vi "eventHardpointActuatorInfo.vi"(8 "error in (no error)":errorcluster, 11 "Publisher in":refnum<class "Publisher.lvclass">) -> (0 "error out":errorcluster, 3 "Publisher out":refnum<class "Publisher.lvclass">)   [LabVIEW 2016, in "Publisher.lvclass"]
uses:
  Publisher.lvclass
  Publisher.lvclass/Publisher.ctl
  UserEvents/UserEvents.lvclass
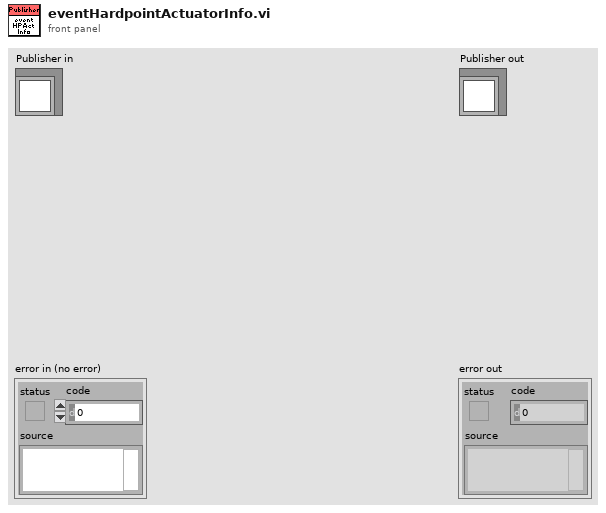
[diagram p1: front panel]
types:
  T1 = typedef "M1M3SupportTopics.lvlib/EventHardpointActuatorInfo.ctl" = cluster{"Timestamp":T2, "ReferenceId":i32[], "ReferencePosition":i32[], "XPosition":sgl[], "YPosition":sgl[], "ZPosition":sgl[], "ILCUniqueId":i64[], "ILCApplicationType":u8[], "NetworkNodeType":u8[], "ILCSelectedOptions":u8[], "NetworkNodeOptions":u8[], "MajorRevision":u8[], "MinorRevision":u8[], "ADCScanRate":u8[], "MainADCCalibrationK1":sgl[], "MainADCCalibrationK2":sgl[], "MainADCCalibrationK3":sgl[], "MainADCCalibrationK4":sgl[], "MainLoadCellOffset":sgl[], "MainLoadCellSensitivity":sgl[], "BackupADCCalibrationK1":sgl[], "BackupADCCalibrationK2":sgl[], "BackupADCCalibrationK3":sgl[], "BackupADCCalibrationK4":sgl[], "BackupLoadCellOffset":sgl[], "BackupLoadCellSensitivity":sgl[], "MainCalibrationError":bool[], "BackupCalibrationError":bool[], "UniqueIdCRCError":bool[], "ApplicationTypeMismatch":bool[], "ApplicationMissing":bool[], "ApplicationCRCMismatch":bool[], "OneWireMissing":bool[], "OneWire1Mismatch":bool[], "OneWire2Mismatch":bool[]}
  T2 = typedef "M1M3SupportTopics.lvlib/Timestamp.ctl" = dbl
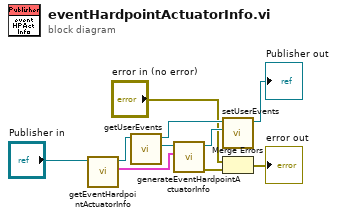
[diagram p0: block diagram]
diagram:
  n1 = call "getEventHardpointActuatorInfo.vi"("Publisher in"="Publisher in") -> ("EventHardpointActuatorInfo"=w1:T1, "Publisher out"=w9:refnum<class "Publisher.lvclass">)  [unwired: 9 in]
  n2 = call "getUserEvents.vi"("Publisher in"=w9) -> ("UserEvents"=w8:refnum<class "UserEvents.lvclass">, "Publisher out"=w6:refnum<class "Publisher.lvclass">)  [unwired: 9 in]
  n3 = call "generateEventHardpointActuatorInfo.vi"("EventHardpointActuatorInfo"=w1, "UserEvents in"=w8) -> ("error out"=w4:errorcluster, "UserEvents out"=w7:refnum<class "UserEvents.lvclass">)  [unwired: 8 in]
  n4 = call "setUserEvents.vi"("UserEvents"=w7, "Publisher in"=w6) -> ("Publisher out"=→"Publisher out":refnum<class "Publisher.lvclass">)  [unwired: 9 in]
  n5 = Merge Errors("error in (no error)", w4) -> (→"error out":errorcluster)
